vi "GetNearestValue.vi"(10 "Value":dbl, 11 "Array":dbl[][](array[numeric])) -> (3 "Nearest Value":dbl)   [LabVIEW 2014, in "Array.lvlib"]
uses:
  Array.lvlib
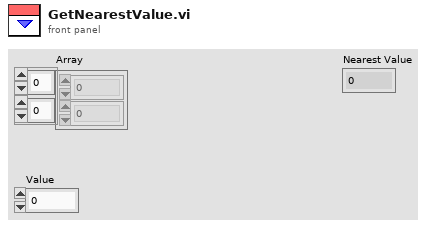
[diagram p1: front panel]
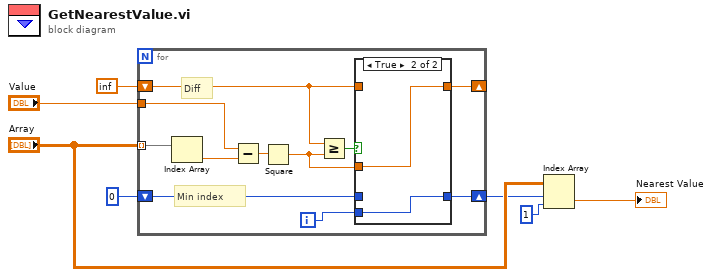
[diagram p0: block diagram]
diagram:
  n1 = for {
    tunnel: "Array" -> [w18] mode=indexing
    tunnel: "Value" -> [w16]
    shift-right: [w14] -> _
    shift-left: inf -> [w10]
    shift-right: [w11] -> w3
    shift-left: 0 -> [w12]
    i -> [w13]
    # "Min index"
    # "Diff"
    n2 = Index Array(array=w18) -> (element=w17:dbl)  [unwired: 1 in]
    n3 = Subtract(x=w16, y=w17) -> (x-y=w15:dbl)
    n4 = Square(x=w15) -> (x^2=w9:dbl)
    n5 = Greater Or Equal?(x=w10, y=w9) -> (x >= y?=w8:bool)
    n6 = case shown="True" w8 {
      tunnel: w10 -> [w20 _]
      tunnel: [w20 w22] -> w14
      tunnel: w9 -> [_ w22]
      tunnel: w13 -> [_ w21]
      tunnel: w12 -> [w19 _]
      tunnel: [w19 w21] -> w11
      frame False {
      }
      frame True {
      }
    }
  }
  n7 = Index Array(array="Array", index (row)=w3, index (col)=1 ("disabled index (col)")) -> (element=→"Nearest Value":dbl)
